vi "IR (SubVI).vi"(8 "error in (no error)":errorcluster, 11 "PWM Ref Out":T1) -> (0 "error out":errorcluster, 3 "Range [cm]":dbl(knob) scale=0.0..80.0)   [LabVIEW 2016]
uses:
  <vilib>/myRIO/Instrument Drivers/Onboard IO/PWM/typedefs/PWM Reference.ctl
  <vilib>/myRIO/Common/Instrument Driver Framework/Utilities/typedefs/myRIO Generic Hardware Reference.ctl
  <vilib>/myRIO/Common/Instrument Driver Framework/Utilities/typedefs/Hardware Version Enum.ctl
  <vilib>/myRIO/Common/Instrument Driver Framework/Utilities/typedefs/myRIO v1.0 Reference.ctl
  <vilib>/myRIO/Common/Instrument Driver Framework/Utilities/typedefs/Generic FPGA Reference.ctl
  <vilib>/myRIO/Common/Instrument Driver Framework/myRIO v1.0/PWM/typedefs/PWM Channels Enum.ctl
  <vilib>/myRIO/Instrument Drivers/Onboard IO/PWM/typedefs/PWM Configuration.ctl
  <vilib>/myRIO/Instrument Drivers/Onboard IO/AI/typedefs/AI Reference.ctl
  <vilib>/myRIO/Common/Instrument Driver Framework/myRIO v1.0/AI/typedefs/AI Channels List.ctl
  <vilib>/myRIO/Common/Instrument Driver Framework/myRIO v1.0/AI/typedefs/AI Channels Enum.ctl
  <vilib>/myRIO/Common/Instrument Driver Framework/Utilities/typedefs/Analog Scaling Constants List.ctl
  <vilib>/myRIO/Common/Instrument Driver Framework/Utilities/typedefs/Analog Scaling Constants.ctl
  <vilib>/userdefined/High Color/nirio_resource_hc.ctl
  <vilib>/myRIO/Common/Instrument Driver Framework/Utilities/vis/Is FPGA Ref Available.vi
  <vilib>/myRIO/Common/Instrument Driver Framework/myRIO v1.0/AI/vis/myRIO v1.1 Open AI.vi
  <vilib>/myRIO/Instrument Drivers/Onboard IO/AI/vis/Read.vi
  <vilib>/myRIO/Common/Instrument Driver Framework/Utilities/vis/Validate Channels.vi
  <vilib>/myRIO/Common/Instrument Driver Framework/myRIO v1.0/AI/vis/myRIO v1.0 Reserve AI.vi
  <vilib>/myRIO/Common/Instrument Driver Framework/myRIO v1.0/AI/vis/myRIO v1.0 Build MUX Configuration AI.vi
  <vilib>/myRIO/Common/Instrument Driver Framework/myRIO v1.0/Resource Manager/vis/myRIO v1.0 Reserve Channel List.vi
  <vilib>/myRIO/Common/Instrument Driver Framework/myRIO v1.0/Resource Manager/vis/myRIO v1.0 Reserve Channel.vi
  <vilib>/myRIO/Common/Instrument Driver Framework/myRIO v1.0/Resource Manager/vis/myRIO v1.0 Unreserve Channel.vi
  <vilib>/myRIO/Common/Instrument Driver Framework/myRIO v1.0/Resource Manager/vis/myRIO v1.0 Build Mutex Name.vi
  <vilib>/Utility/error.llb/Error Cluster From Error Code.vi
  <vilib>/myRIO/Common/Instrument Driver Framework/myRIO v1.0/PWM/vis/myRIO v1.0 Write PWM.vi
  <vilib>/Utility/VariantDataType/GetNumericInfo.vi
  <vilib>/myRIO/Common/Instrument Driver Framework/myRIO v1.0/myRIO v1.1 Open.vi
  <vilib>/myRIO/Common/Instrument Driver Framework/myRIO v1.0/AI/vis/myRIO v1.0 Get Scaling Constants AI.vi
  <vilib>/myRIO/Common/Instrument Driver Framework/Utilities/vis/IO Manager.vi
  <vilib>/myRIO/Common/Instrument Driver Framework/Utilities/vis/Configuration Manager.vi
  <vilib>/myRIO/Common/Instrument Driver Framework/myRIO v1.0/myRIO v1.0 Close.vi
  <vilib>/myRIO/Common/Instrument Driver Framework/myRIO v1.0/AI/vis/myRIO v1.0 Read AI.vi
  <vilib>/myRIO/Express VI/Onboard IO/AI/AI Express VI.xnode
  <vilib>/myRIO/Instrument Drivers/Onboard IO/AI/vis/myRIO AI Open.xnode
  <vilib>/ptbypt/NI_PtbyPt.lvlib
  <vilib>/myRIO/Instrument Drivers/Onboard IO/AI/AI.lvlib
  <vilib>/myRIO/Instrument Drivers/Onboard IO/PWM/PWM.lvlib
panel:
  in  "ESC":bool
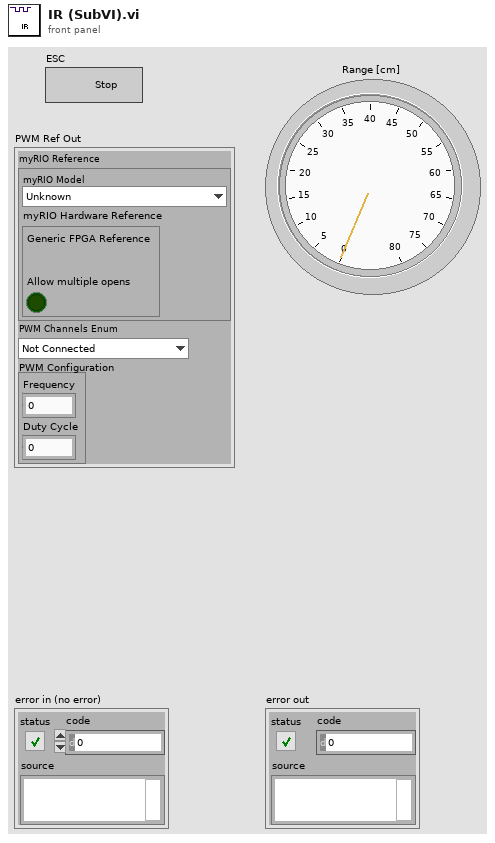
[diagram p1: front panel]
types:
  T1 = typedef "PWM.lvlib/PWM Reference.ctl" = cluster{"myRIO Reference":T2, "PWM Channels Enum":T6, "PWM Configuration":T7}
  T2 = typedef "myRIO Generic Hardware Reference.ctl" = cluster{"myRIO Model":T3, "myRIO Hardware Reference":T4}
  T3 = typedef "Hardware Version Enum.ctl" = enum16{"Unknown", "myRIO-1900", "myRIO-1950", "roboRIO", "NI ELVIS RIO CM"}
  T4 = typedef "myRIO v1.0 Reference.ctl" = cluster{"Generic FPGA Reference":T5, "Allow multiple opens":bool}
  T5 = typedef "Generic FPGA Reference.ctl" = refnum<k20>
  T6 = typedef "PWM Channels Enum.ctl" = enum16{"Not Connected", "C/PWM0", "C/PWM1", "A/PWM0", "A/PWM1", "A/PWM2", "B/PWM0", "B/PWM1", "B/PWM2", "PWM/PWM0", "PWM/PWM1", "PWM/PWM2", "PWM/PWM3", "PWM/PWM4", "PWM/PWM5", "PWM/PWM6", "PWM/PWM7", "PWM/PWM8", "PWM/PWM9"}
  T7 = typedef "PWM.lvlib/PWM Configuration.ctl" = cluster{"Frequency":dbl, "Duty Cycle":dbl}
  T8 = typedef "AI.lvlib/AI Reference.ctl" = cluster{"myRIO Reference":T2, "AI Channels List":T9, "AI Scaling Constants List":T11}
  T9 = typedef "AI Channels List.ctl" = T10[]
  T10 = typedef "AI Channels Enum.ctl" = enum16{"Not Connected", "AudioIn/Left", "AudioIn/Right", "C/AI0", "C/AI1", "A/AI0", "A/AI1", "A/AI2", "A/AI3", "B/AI0", "B/AI1", "B/AI2", "B/AI3", "AI/AI0", "AI/AI1", "AI/AI2", "AI/AI3"}
  T11 = typedef "Analog Scaling Constants List.ctl" = T12[]
  T12 = typedef "Analog Scaling Constants.ctl" = cluster{"LSB Weight (Volts)":dbl, "Offset (Volts)":dbl, "Signed?":bool}
  T13 = typedef "nirio_resource_hc.ctl" = tag
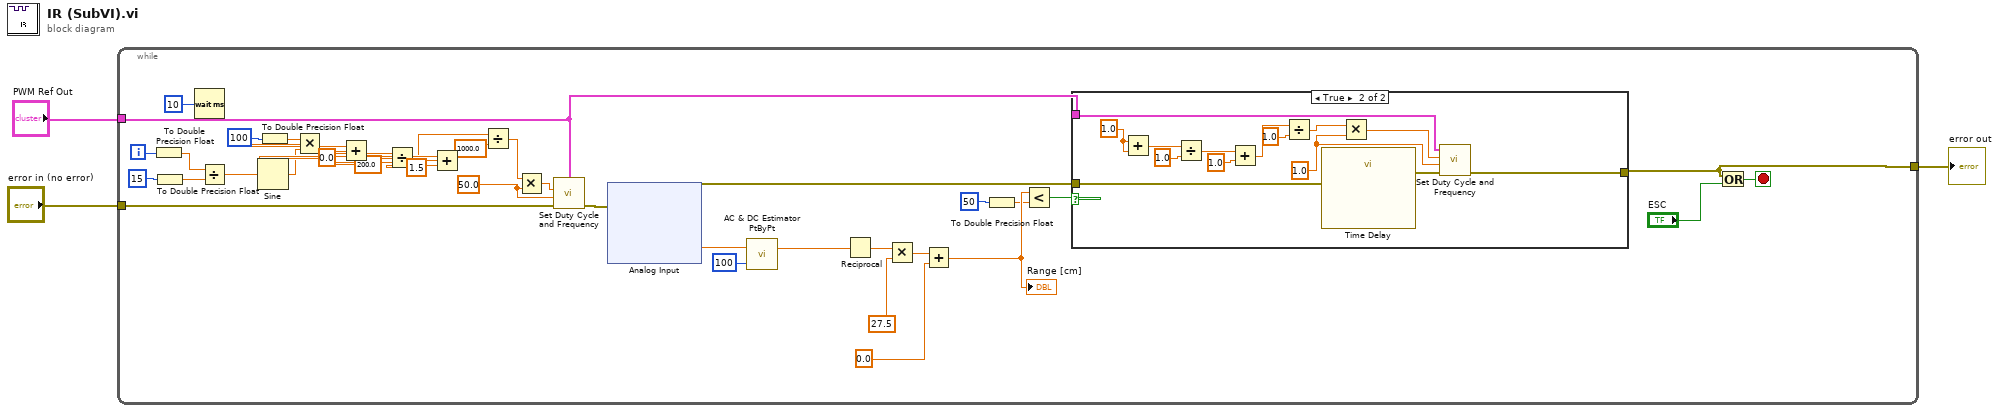
[diagram p0: block diagram]
diagram:
  n1 = while {
    tunnel: [w11] -> w3
    tunnel: "error in (no error)" -> [w22]
    tunnel: "PWM Ref Out" -> [w5]
    i -> [w17]
    stop <- w40 stop-if-true
    w25 = 50.0 ("freq [Hz] in")
    n2 = To Double Precision Float(number=w17) -> (double precision float=w7:dbl)
    n3 = To Double Precision Float(number=15) -> (double precision float=w8:dbl)
    n4 = Wait (ms)(milliseconds to wait=u32 10) -> ()  [unwired: 1 out]
    n5 = Divide(x=w7, y=w8) -> (x/y=w18:dbl)
    n6 = Sine(x=w18) -> (sin(x)=w21:dbl)
    n7 = To Double Precision Float(number=100) -> (double precision float=w6:dbl)
    n8 = Multiply(x=w6, y=w21) -> (x*y=w16:dbl)
    n9 = Add(x=w16, y=0.0 ("position [%FS]")) -> (x+y=w28:dbl)
    n10 = Divide(x=w28, y=200.0) -> (x/y=w32:dbl)
    n11 = Add(x=w32, y=1.5) -> (x+y=w30:dbl)
    n12 = Divide(x=w30, y=1000.0) -> (x/y=w27:dbl)
    n13 = Multiply(x=w27, y=w25) -> (x*y=w26:dbl)
    n14 = call <vilib>:"Set Duty Cycle and Frequency.vi"("error in (no error)"=w22, "Frequency [Hz]"=w25, "Duty Cycle"=w26, "PWM Ref In"=w5) -> ("error out"=w23:errorcluster)  [unwired: 5 in, 1 out]
    n15 = xnode "Analog Input"("error in (no error)"=w23) -> ("B/AI0 (Pin 3)"=w10:dbl, "error out"=w12:errorcluster)
    n16 = call <vilib>:"AC & DC Estimator PtByPt.vi"("signal"=w10, "sample length"=100) -> ("DC estimate (V)"=w37:dbl)  [unwired: 1 in, 2 out]
    n17 = Reciprocal(x=w37) -> (1/x=w39:dbl)
    n18 = Multiply(x=w39, y=27.5 ("Kscale [cm-V]")) -> (x*y=w34:dbl)
    n19 = Add(x=w34, y=0.0 ("Koffset [cm]")) -> (x+y=w14:dbl)
    "Range [cm]" <- w14
    n20 = To Double Precision Float(number=50) -> (double precision float=w9:dbl)
    n21 = Less?(x=w14, y=w9) -> (x < y?=w15:bool)
    n22 = case shown="True" w15 {
      tunnel: w5 -> [_ w47]
      tunnel: w12 -> [w42 w44]
      tunnel: [w42 w45] -> w11
      frame False {
      }
      frame True {
        w46 = 1.0
        w48 = 1.0 ("position [%FS]")
        n23 = Add(x=w48, y=w48) -> (x+y=w51:dbl)
        n24 = Divide(x=w51, y=1.0) -> (x/y=w55:dbl)
        n25 = Add(x=w55, y=1.0) -> (x+y=w53:dbl)
        n26 = Divide(x=w53, y=1.0) -> (x/y=w50:dbl)
        n27 = call "Time Delay"("error in (no error)"=w44) -> ("error out"=w43:errorcluster)  [unwired: 10 in]
        n28 = Multiply(x=w50, y=w46) -> (x*y=w49:dbl)
        n29 = call <vilib>:"Set Duty Cycle and Frequency.vi"("error in (no error)"=w43, "Frequency [Hz]"=w46, "Duty Cycle"=w49, "PWM Ref In"=w47) -> ("error out"=w45:errorcluster)  [unwired: 5 in, 1 out]
      }
    }
    n30 = Or(x=w11, y="ESC") -> (x .or. y?=w40:bool)
  }
  "error out" <- w3
